vi "PAN_TCPSERVER_Create.vi"(4 "log":bool, 6 "logfile":path, 8 "error in (no error)":errorcluster, 10 "port":u16, 11 "messages from socks Q name":string) -> (0 "error out":errorcluster, 2 "queue out":refnum<queue>, 3 "listener ID":refnum<k5>)   [LabVIEW 2016]
uses:
  private/vis/PAN_TCPSERVER_MsgStruct.ctl
panel:
  in  "ResponseStruct":T1
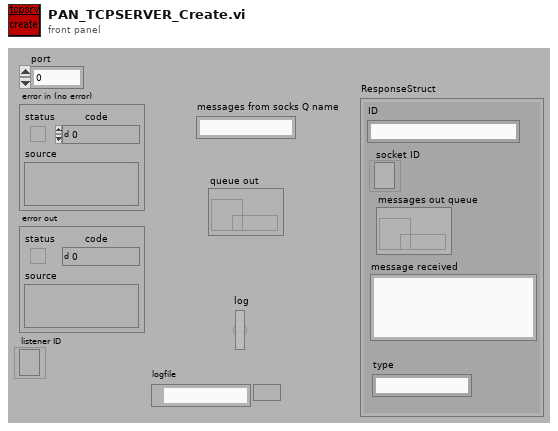
[diagram p1: front panel]
types:
  T1 = typedef "PAN_TCPSERVER_MsgStruct.ctl" = cluster{"ID":string, "socket ID":refnum<k5>, "messages out queue":refnum<queue>, "message received":string, "type":string}
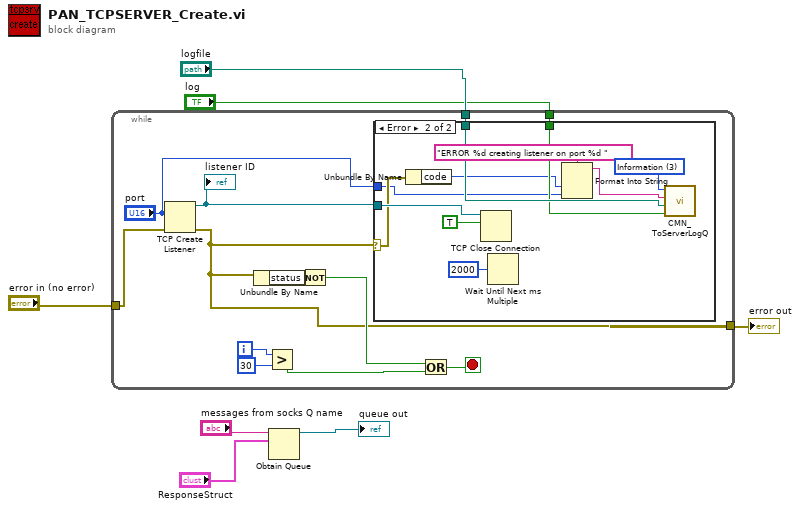
[diagram p0: block diagram]
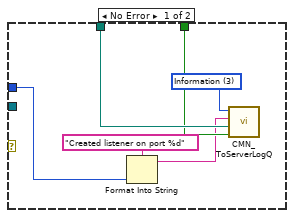
[diagram p2: hidden frame]
diagram:
  n1 = while {
    tunnel: "error in (no error)" -> [w12]
    tunnel: [w11] -> w3
    tunnel: "logfile" -> [w10]
    tunnel: "log" -> [w9]
    i -> [w16]
    stop <- w17 stop-if-true
    n2 = TCP Create Listener(8:w12, 10:"port") -> (0:w11:errorcluster, 3:w13:refnum<k5>)  [unwired: 4 out]
    "listener ID" <- w13
    n3 = Unbundle By Name(w11) -> ("status"=w19:bool)
    n4 = Greater?(x=w16, y=30) -> (0:w14:bool)
    n5 = Not(x=w19) -> (.not. x?=w18:bool)
    n6 = case shown="Error" w11 {
      selector: w11 -> [_ w29]
      tunnel: w13 -> [_ w35]
      tunnel: w10 -> [w25 w32]
      tunnel: w9 -> [w24 w31]
      tunnel: "port" -> [w21 w27]
      frame No Error {
        w23 = u16 3 items=["command", "imediateReply", "Callback Reply", "Information", "none"] ("type")
        n7 = Format Into String(format string="Created listener on port %d", w21) -> (resulting string=w20:string)  [unwired: 2 in, 1 out]
        n8 = call "CMN_ToServerLogQ.vi"("Log"=w24, "file"=w25, "string"=w20, "type"=w23) -> ()  [unwired: 2 in, 5 out]
      }
      frame Error {
        w33 = u16 3 items=["command", "imediateReply", "Callback Reply", "Information", "none"] ("type")
        n9 = Unbundle By Name(w29) -> ("code"=w28:i32)
        n10 = TCP Close Connection(connection ID=w35, abort (F)=TRUE) -> ()  [unwired: 1 in, 2 out]
        n11 = Wait Until Next ms Multiple(millisecond multiple=u32 2000) -> ()  [unwired: 1 out]
        n12 = Format Into String(format string="ERROR %d creating listener on port %d ", w28, w27) -> (resulting string=w26:string)  [unwired: 2 in, 1 out]
        n13 = call "CMN_ToServerLogQ.vi"("Log"=w31, "file"=w32, "string"=w26, "type"=w33) -> ()  [unwired: 2 in, 5 out]
      }
    }
    n14 = Or(x=w18, y=w14) -> (x .or. y?=w17:bool)
  }
  "error out" <- w3
  n15 = Obtain Queue(name (unnamed)="messages from socks Q name", element data type="ResponseStruct") -> (queue out=→"queue out":refnum<queue>)  [unwired: 3 in, 2 out]
